vi "BuildDrvInfo.vi"(5 "Camera in":refnum<class "CameraI2COUSB.lvclass">) -> (0 "Camera out":refnum<class "CameraI2COUSB.lvclass">, 2 "Lib Path":path, 3 "Class Name":string)   [LabVIEW 2020, in "CameraI2COUSB.lvlib" / "CameraI2COUSB.lvclass"]
uses:
  CameraI2COUSB.lvclass
  CameraI2COUSB.lvclass/CameraI2COUSB.ctl
panel:
  out "error out":errorcluster
  in  "error in (no error)":errorcluster
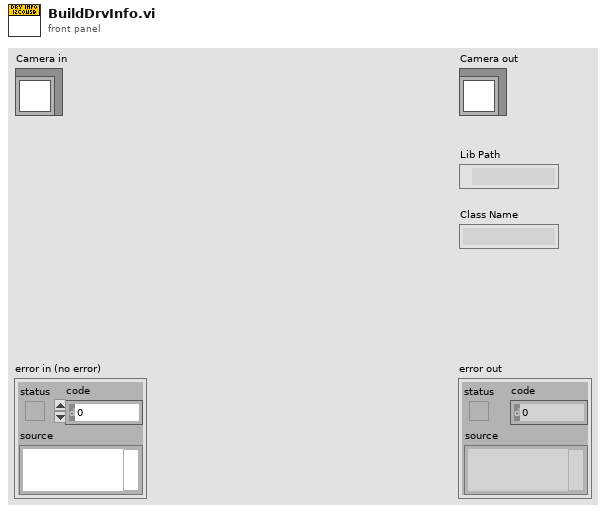
[diagram p1: front panel]
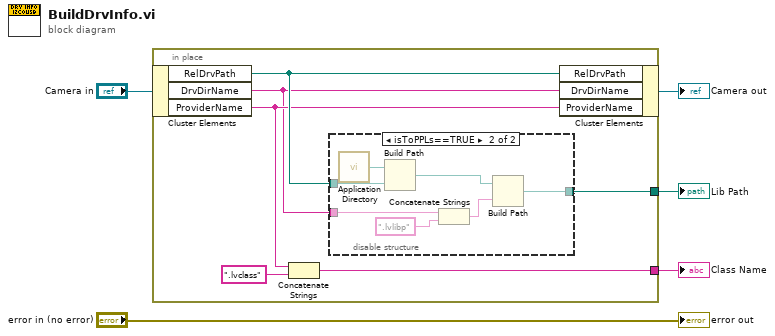
[diagram p0: block diagram]
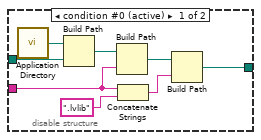
[diagram p2: hidden frame]
diagram:
  n1 = in-place {
    in-place-border: [w11] -> w2
    in-place-border: [w7] -> w1
    n2 = in-place-cluster #1("Camera in") -> ("RelDrvPath"=w9:path, "DrvDirName"=w6:string, "ProviderName"=w8:string)
    n3 = Concatenate Strings(w8, ".lvclass" ("y")) -> (w7:string)
    n4 = disable-structure shown="isToPPLs==TRUE" {
      disable-tunnel: [w14 w22] -> w11
      disable-tunnel: w9 -> [w13 w21]
      disable-tunnel: w6 -> [w12 w20]
      frame condition #0 (active) {
        n5 = call <vilib>:"Application Directory.vi"() -> ("Application Directory"=w18:path)
        n6 = Build Path(base path=w18, name or relative path=w13) -> (appended path=w19:path)
        n7 = Build Path(base path=w19, name or relative path=w12) -> (appended path=w16:path)
        n8 = Concatenate Strings(w12, ".lvlib") -> (w15:string)
        n9 = Build Path(base path=w16, name or relative path=w15) -> (appended path=w14:path)
      }
      frame condition #1 {
        n10 = call <vilib>:"Application Directory.vi"() -> ("Application Directory"=w25:path)
        n11 = Build Path(base path=w25, name or relative path=w21) -> (appended path=w26:path)
        n12 = Concatenate Strings(w20, ".lvlibp") -> (w23:string)
        n13 = Build Path(base path=w26, name or relative path=w23) -> (appended path=w22:path)
      }
    }
    n14 = in-place-cluster #1("RelDrvPath"=w9, "DrvDirName"=w6, "ProviderName"=w8) -> (→"Camera out":refnum<class "CameraI2COUSB.lvclass">)
  }
  "Class Name" <- w1
  "Lib Path" <- w2
  "error out" <- "error in (no error)"
